vi "Send.vi"(8 "error in (no error)":errorcluster, 10 "Message":refnum<class "MSG.lvclass">, 11 "NotifierMessenger in":refnum<class "NotifierMessenger.lvclass">) -> (0 "error out":errorcluster, 3 "NotifierMessenger out":refnum<class "NotifierMessenger.lvclass">)   [LabVIEW 2011, in "Messenging.lvlib" / "NotifierMessenger.lvclass"]
uses:
  NotifierMessenger.lvclass
  TextVarientMessage/MSG.lvclass
  NotifierMessenger.lvclass/NotifierMessenger.ctl
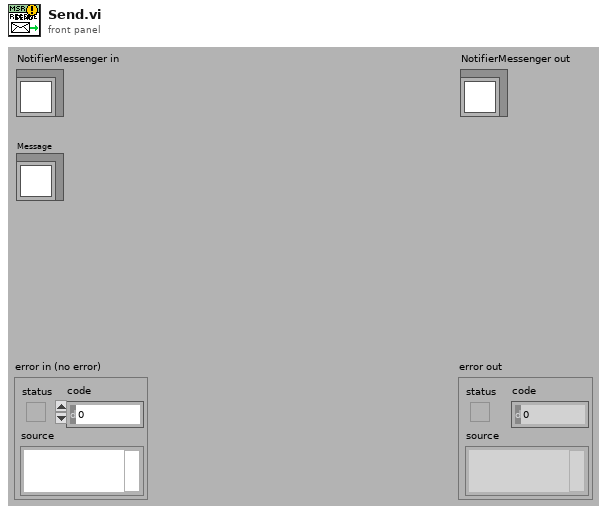
[diagram p1: front panel]
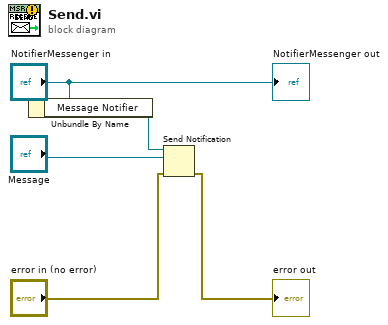
[diagram p0: block diagram]
diagram:
  n1 = Unbundle By Name("NotifierMessenger in") -> ("Message Notifier"=w4:refnum<notifier>)
  n2 = Send Notification(notification="Message", notifier=w4, error in (no error)="error in (no error)") -> (error out=→"error out":errorcluster)  [unwired: 1 out]
  "NotifierMessenger out" <- "NotifierMessenger in"
